vi "Wait for Response.vi"(8 "error in (no error)":errorcluster, 9 "Timeout (-1)":i32=-1, 10 "id String":string, 11 "JSONRPC Server in":refnum<class "JSONRPC Server.lvclass">) -> (0 "error out":errorcluster, 2 "JSON Response String":string, 3 "JSONRPC Server out":refnum<class "JSONRPC Server.lvclass">)   [LabVIEW 2015, in "JSONRPC Server.lvclass"]
doc: "This blocks until a Response with the given id is found on the RPC Server."
uses:
  JSONRPC Server.lvclass
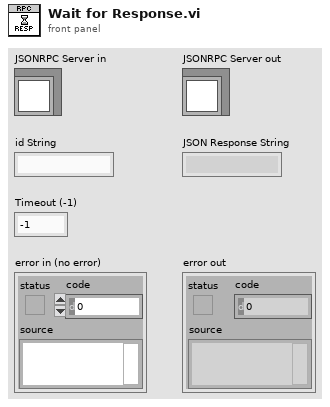
[diagram p1: front panel]
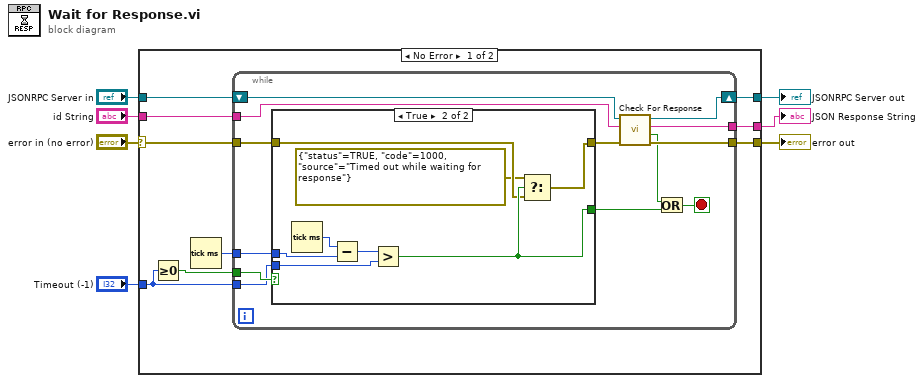
[diagram p0: block diagram]
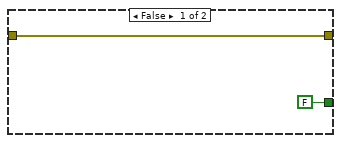
[diagram p2: hidden frame]
diagram:
  n1 = case shown="No Error" "error in (no error)" {
    selector: "error in (no error)" -> [w12 w41]
    tunnel: [w11 w41] -> w6
    tunnel: [w15 w40] -> w4
    tunnel: "JSONRPC Server in" -> [w16 w40]
    tunnel: "id String" -> [w13 _]
    tunnel: "Timeout (-1)" -> [w8 _]
    tunnel: [w14 _] -> w1
    frame No Error {
      n2 = Greater Or Equal To 0?(x=w8) -> (x >= 0?=w10:bool)
      n3 = Tick Count (ms)() -> (millisecond timer value=w9:u32)
      n4 = while {
        shift-right: [w28] -> w15
        shift-left: w16 -> [w29]
        tunnel: [w27] -> w14
        tunnel: w13 -> [w26]
        tunnel: w12 -> [w18]
        tunnel: [w25] -> w11
        tunnel: w10 -> [w24]
        tunnel: w9 -> [w23]
        tunnel: w8 -> [w22]
        stop <- w19 stop-if-true
        n5 = case shown="True" w24 {
          tunnel: w23 -> [_ w38]
          tunnel: w22 -> [_ w36]
          tunnel: [FALSE w35] -> w21
          tunnel: w18 -> [w30 w34]
          tunnel: [w30 w33] -> w17
          frame False {
          }
          frame True {
            n6 = Tick Count (ms)() -> (millisecond timer value=w39:u32)
            n7 = Subtract(x=w39, y=w38) -> (x-y=w37:u32)
            n8 = Greater?(x=w37, y=w36) -> (0:w35:bool)
            n9 = Select(t=errorcluster {"status"=TRUE, "code"=1000, "source"="Timed out while waiting for response"}, s=w35, f=w34) -> (s? t:f=w33:errorcluster)
          }
        }
        n10 = call-dynamic "Check For Response.vi"("error in (no error)"=w17, "id String"=w26, "Server in"=w29) -> ("error out"=w25:errorcluster, "found"=w20:bool, "response string"=w27:string, "Server out"=w28:refnum<class "JSONRPC Server.lvclass">)  [unwired: 5 in]
        n11 = Or(x=w20, y=w21) -> (x .or. y?=w19:bool)
      }
    }
    frame Error {
    }
  }
  "error out" <- w6
  "JSONRPC Server out" <- w4
  "JSON Response String" <- w1
